vi "Test DMAC Conversion.vi"() -> ()   [LabVIEW 2021]
uses:
  <vilib>/Utility/error.llb/Trim Whitespace.vi
  Networking_CIF_U.lvlib
panel:
  out "Pass":bool
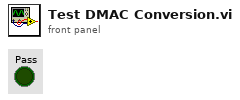
[diagram p1: front panel]
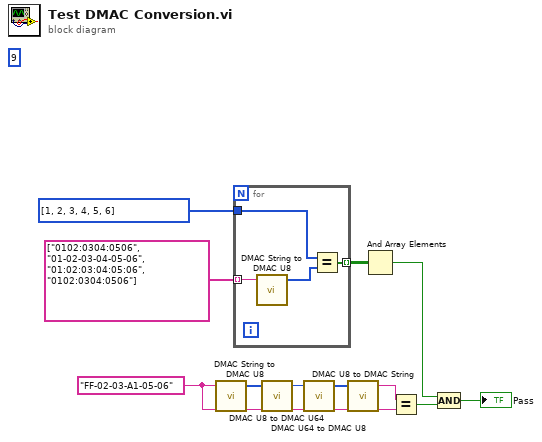
[diagram p0: block diagram]
diagram:
  w4 = "FF-02-03-A1-05-06" ("DMAC String")
  (unwired) 9
  n1 = call "DMAC String to DMAC U8.vi"("DMAC String"=w4) -> ("DestinationMACAddress"=w8:u8[])  [unwired: 4 in]
  n2 = for {
    tunnel: string[] ["0102:0304:0506", "01-02-03-04-05-06", "01:02:03:04:05:06", "0102:0304:0506"] -> [w15] mode=indexing
    tunnel: u8[] [1, 2, 3, 4, 5, 6] ("DestinationMACAddress  2") -> [w13]
    tunnel: [w12] -> w9 mode=indexing
    n3 = call "DMAC String to DMAC U8.vi"("DMAC String"=w15) -> ("DestinationMACAddress"=w14:u8[])  [unwired: 4 in]
    n4 = Equal?(x=w13, y=w14) -> (x = y?=w12:bool[])
  }
  n5 = call "DMAC U8 to DMAC U64.vi"("DestinationMACAddress"=w8) -> ("DMAC U64"=w7:u64)  [unwired: 4 in]
  n6 = call "DMAC U64 to DMAC U8.vi"("DMAC U64"=w7) -> ("DestinationMACAddress"=w6:u8[])  [unwired: 4 in]
  n7 = call "DMAC U8 to DMAC String.vi"("DestinationMACAddress"=w6) -> ("DMAC String"=w5:string)  [unwired: 4 in]
  n8 = And Array Elements(Boolean array=w9) -> (logical AND=w2:bool)
  n9 = Equal?(x=w5, y=w4) -> (x = y?=w1:bool)
  n10 = Compound Arithmetic op=AND(w2, w1) -> (→"Pass":bool)
